vi "generate_pcode.vi"(7 "ParticipantID":string, 10 "Direction":bool=TRUE, 11 "number":i32) -> (3 "Code":string)   [LabVIEW 2018]
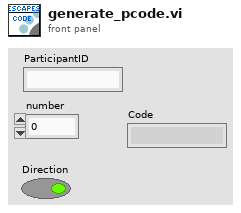
[diagram p1: front panel]
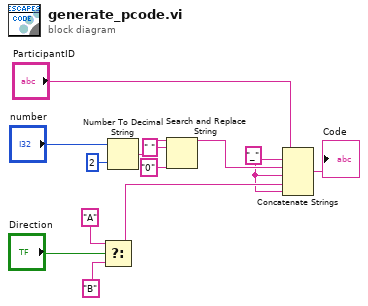
[diagram p0: block diagram]
diagram:
  w1 = "_" ("Filename")
  n1 = Select(t="A" ("replace string (\"\")"), s="Direction", f="B" ("replace string (\"\")")) -> (s? t:f=w2:string)
  n2 = Number To Decimal String(number="number", width (-)=i16 2) -> (decimal integer string=w11:string)
  n3 = Search and Replace String(input string=w11, search string=" ", replace string="0" ("replace string (\"\")")) -> (result string=w8:string)  [unwired: 5 in, 3 out]
  n4 = Concatenate Strings("ParticipantID", w1, w8, w1, w2, w1) -> (→"Code":string)
